vi "Keithley DMM6500 DAQ6500 Series Grading and Binning Resistors.vi"() -> ()   [LabVIEW 2023]
doc: "This example shows how to configure Grading and Binning Resistors trigger."
uses:
  <instrlib>/Keithley DMM6500 DAQ6500 Series/Keithley DMM6500 DAQ6500 Series.lvlib
panel:
  in  "Arguments ()":string="100, 5, .1, .1, 120, 80, 15, 4, 110, 90, 1, 105, 95, 2, 101, 99, 3,\"bufferVar\""
  in  "Buffer Name (\"bufferVar\")":string="bufferVar"
  in  "Buffer Size (10)":u32=1000000
  in  "VISA resource name":refnum<visa-resource-name>
  # "(c) 2018-2022 National Instruments.  ALL RIGHTS RESERVED."
  # "This VI example demonstrates how to use the DMM6500 or DAQ6500 Series to\n perform benchtop binning operations using one of the instrument's predefined\n trigger models, GradeBinning, to control external component-handling devices \nwith digital I/O. This resistance grading application uses limit tests to inspect a\nsingle resistor under test against multiple limits until the first failure occurs."
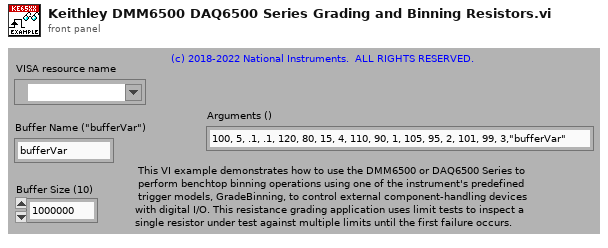
[diagram p1: front panel]
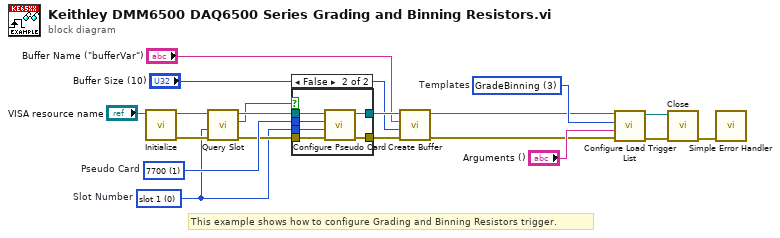
[diagram p0: block diagram]
diagram:
  w1 = 0 items=["slot 1", "slot 2"]  # Slot Number
  w7 = 1 items=["0", "7700", "7701", "7702", "7703", "7705", "7706", "7707", "7708", "7709", "7710", "7711", "7712"]  # Pseudo Card
  w11 = 3 items=["ConfigList", "DurationLoop", "Empty", "GradeBinning", "Keithley2001", "LogicTrigger", "LoopUntilEvent", "SimpleLoop", "SortBinning"]  # Templates
  # "This example shows how to configure Grading and Binning Resistors trigger."
  n1 = call <instrlib>:"Initialize.vi"("VISA resource name"="VISA resource name") -> ("error out"=w4:errorcluster, "VISA resource name out"=w6:refnum<visa-resource-name>)  [unwired: 9 in]
  n2 = call <instrlib>:"Query Slot.vi"("error in (no error)"=w4, "Slot Number(0: slot 1)"=w1, "VISA resource name"=w6) -> ("error out"=w3:errorcluster, "Real Card In Slot"=w2:bool, "VISA resource name out"=w5:refnum<visa-resource-name>)  [unwired: 6 in]
  n3 = case shown="False" w2 {
    tunnel: [w21 w27] -> w17
    tunnel: [w20 w26] -> w16
    tunnel: w7 -> [_ w25]
    tunnel: w1 -> [_ w24]
    tunnel: w5 -> [w21 w23]
    tunnel: w3 -> [w20 w22]
    frame True {
    }
    frame False {
      n4 = call <instrlib>:"Configure Pseudo Card.vi"("error in (no error)"=w22, "Slot Number (0: slot1)"=w24, "Pseudo Card (0:No pseudocard)"=w25, "VISA resource name"=w23) -> ("error out"=w26:errorcluster, "VISA resource name out"=w27:refnum<visa-resource-name>)  [unwired: 6 in]
    }
  }
  n5 = call <instrlib>:"Create Buffer.vi"("error in (no error)"=w16, "Buffer Size (10)"="Buffer Size (10)", "Buffer Name (\"\")"="Buffer Name (\"bufferVar\")", "VISA resource name"=w17) -> ("error out"=w8:errorcluster, "VISA resource name out"=w9:refnum<visa-resource-name>)  [unwired: 6 in]
  n6 = call <instrlib>:"Configure Load Trigger List.vi"("error in (no error)"=w8, "ConfigList (MEASURE_LIST)"="Arguments ()", "Templates (0: ConfigList)"=w11, "VISA resource name"=w9) -> ("error out"=w12:errorcluster, "VISA resource name out"=w13:refnum<visa-resource-name>)  [unwired: 6 in]
  n7 = call <instrlib>:"Close.vi"("error in (no error)"=w12, "VISA resource name"=w13) -> ("error out"=w19:errorcluster)  [unwired: 9 in]
  n8 = call <vilib>:"Simple Error Handler.vi"("error in (no error)"=w19) -> ()  [unwired: 4 in, 5 out]
